vi "Convert Received String to Data.vi"(4 "String":string) -> (1 "Cluster":T1, 2 "Data":string[](array[string]))   [LabVIEW 2019]
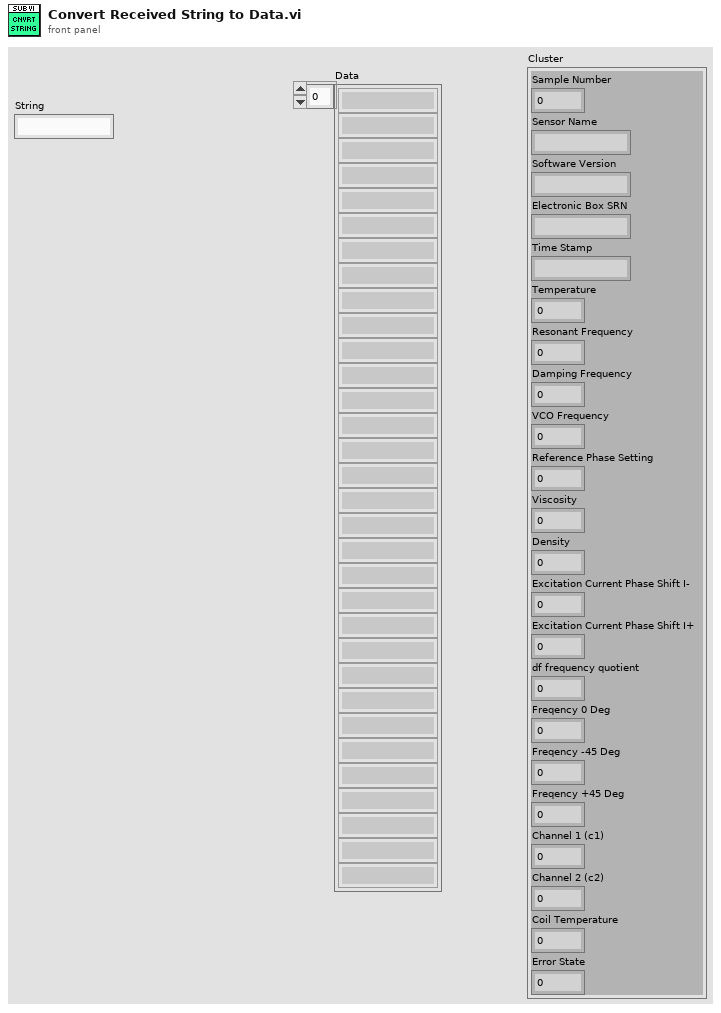
[diagram p1: front panel]
types:
  T1 = cluster{"Sample Number":u16, "Sensor Name":string, "Software Version":string, "Electronic Box SRN":string, "Time Stamp":string, "Temperature":dbl, "Resonant Frequency":dbl, "Damping Frequency":dbl, "VCO Frequency":u16, "Reference Phase Setting":u16, "Viscosity":dbl, "Density":dbl, "Excitation Current Phase Shift I-":u16, "Excitation Current Phase Shift I+":u16, "df frequency quotient":dbl, "Freqency 0 Deg":dbl, "Freqency -45 Deg":dbl, "Freqency +45 Deg":dbl, "Channel 1 (c1)":dbl, "Channel 2 (c2)":dbl, "Coil Temperature":dbl, "Error State":u8}
  T2 = cluster{u16, "String":string, "String":string, "String":string, "date/time string":string, "String":dbl, "String":dbl, "String":dbl, u16, u16, "String":dbl, "String":dbl, u16, u16, "String":dbl, "String":dbl, "String":dbl, "String":dbl, "String":dbl, "String":dbl, "String":dbl, u8}
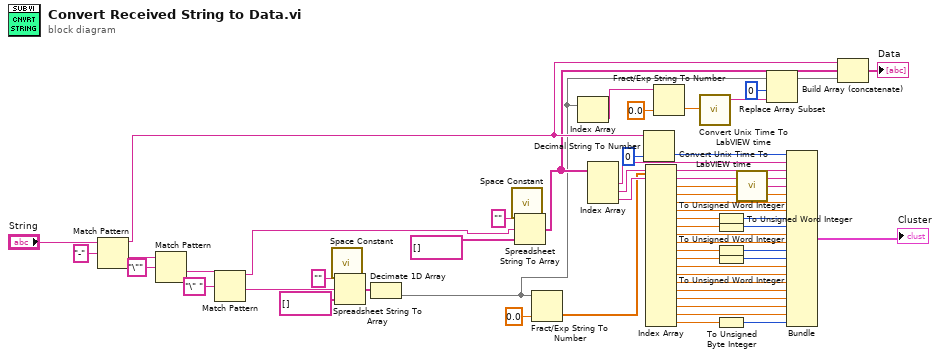
[diagram p0: block diagram]
diagram:
  n1 = Match Pattern(string="String", regular expression="-") -> (before substring=w11:string, after substring=w16:string)  [unwired: 1 in, 2 out]
  n2 = Match Pattern(string=w16, regular expression="\"") -> (after substring=w20:string)  [unwired: 1 in, 3 out]
  n3 = Match Pattern(string=w20, regular expression="\" ") -> (before substring=w26:string, after substring=w21:string)  [unwired: 1 in, 2 out]
  n4 = call <vilib>:"Space Constant.vi"() -> ("String"=w14:string)
  n5 = Spreadsheet String To Array(delimiter (Tab)=w14, format string="", spreadsheet string=w21, array type (2D Dbl)=string[] []) -> (array=w22:string[])
  n6 = Decimate 1D Array(w22) -> (w9:string[])  [unwired: 1 out]
  n7 = call <vilib>:"Space Constant.vi"() -> ("String"=w23:string)
  n8 = Spreadsheet String To Array(delimiter (Tab)=w23, format string="", spreadsheet string=w26, array type (2D Dbl)=string[] []) -> (array=w10:string[])
  n9 = Fract/Exp String To Number(string=w9, default (0 dbl)=0.0 ("default (0 DBL)")) -> (number=w28:dbl[])  [unwired: 2 in, 1 out]
  n10 = Index Array(array=w9) -> (element=w7:string)  [unwired: 1 in]
  n11 = Index Array(array=w10) -> (element #1=w31:string, element #2=w32:string, element #3=w33:string)  [unwired: 3 in]
  n12 = Decimal String To Number(string=w11, default (0L)=u16 0 ("default (0 I32)")) -> (number=w29:u16)  [unwired: 1 in, 1 out]
  n13 = Index Array(array=w28) -> (element #1=w34:dbl, element #2=w36:dbl, element #3=w37:dbl, element #4=w38:dbl, element #5=w39:dbl, element #6=w40:dbl, element #7=w41:dbl, element #8=w42:dbl, element #9=w43:dbl, element #10=w44:dbl, element #11=w45:dbl, element #12=w46:dbl, element #13=w47:dbl, element #14=w48:dbl, element #15=w49:dbl, element #16=w50:dbl, element #17=w51:dbl, element #18=w52:dbl)  [unwired: 18 in]
  n14 = Fract/Exp String To Number(string=w7, default (0 dbl)=0.0 ("default (0 DBL)")) -> (number=w6:dbl)  [unwired: 2 in, 1 out]
  n15 = call "Convert Unix Time To LabVIEW time.vi"("String"=w6) -> ("date/time string"=w4:string)  [unwired: 6 in]
  n16 = To Unsigned Word Integer(number=w39) -> (unsigned 16bit integer=w53:u16)
  n17 = To Unsigned Word Integer(number=w40) -> (unsigned 16bit integer=w54:u16)
  n18 = To Unsigned Word Integer(number=w43) -> (unsigned 16bit integer=w55:u16)
  n19 = To Unsigned Word Integer(number=w44) -> (unsigned 16bit integer=w56:u16)
  n20 = To Unsigned Byte Integer(number=w52) -> (unsigned 8bit integer=w57:u8)
  n21 = call "Convert Unix Time To LabVIEW time.vi"("String"=w34) -> ("date/time string"=w35:string)  [unwired: 6 in]
  n22 = Replace Array Subset(array=w9, new element=w4, index=0) -> (w5:string[])
  n23 = Bundle(w29, "String"=w31, "String"=w32, "String"=w33, "date/time string"=w35, "String"=w36, "String"=w37, "String"=w38, w53, w54, "String"=w41, "String"=w42, w55, w56, "String"=w45, "String"=w46, "String"=w47, "String"=w48, "String"=w49, "String"=w50, "String"=w51, w57) -> (→"Cluster":T2)  [unwired: 1 in]
  n24 = Build Array (concatenate)(w11, w10, w5) -> (→"Data":string[])
